vi "Row-Col Average for 2D array.vi"(10 "2D Array":dbl[][](array[numeric])) -> (1 "Column Averages":dbl[](array[numeric]), 2 "Row Averages":dbl[](array[numeric]))   [LabVIEW 2018]
panel:
  out "Total Array Average":dbl
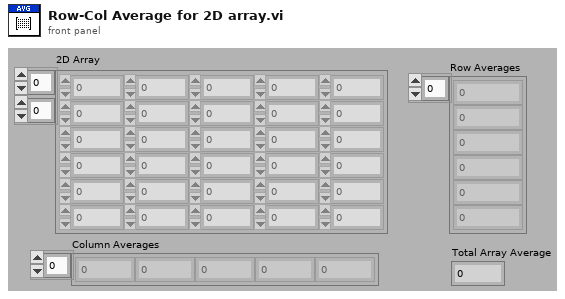
[diagram p1: front panel]
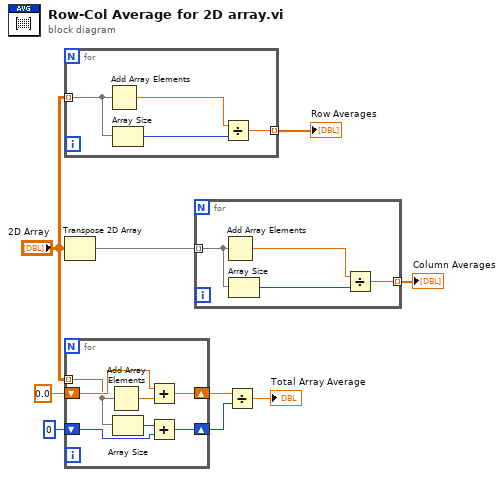
[diagram p0: block diagram]
diagram:
  n1 = for {
    tunnel: "2D Array" -> [w10] mode=indexing
    tunnel: [w12] -> w9 mode=indexing
    n2 = Add Array Elements(numeric array=w10) -> (sum=w13:dbl)
    n3 = Array Size(array=w10) -> (size(s)=w11:i32)
    n4 = Divide(x=w13, y=w11) -> (x/y=w12:dbl)
  }
  "Row Averages" <- w9
  n5 = Transpose 2D Array(2D array="2D Array") -> (transposed array=w8:dbl[][])
  n6 = for {
    tunnel: "2D Array" -> [w17] mode=indexing
    shift-right: [w18] -> w4
    shift-left: 0.0 -> [w20]
    shift-right: [w15] -> w3
    shift-left: 0 -> [w14]
    n7 = Add Array Elements(numeric array=w17) -> (sum=w19:dbl)
    n8 = Array Size(array=w17) -> (size(s)=w16:i32)
    n9 = Add(x=w20, y=w19) -> (x+y=w18:dbl)
    n10 = Add(x=w16, y=w14) -> (x+y=w15:i32)
  }
  n11 = for {
    tunnel: w8 -> [w22] mode=indexing
    tunnel: [w23] -> w7 mode=indexing
    n12 = Add Array Elements(numeric array=w22) -> (sum=w24:dbl)
    n13 = Array Size(array=w22) -> (size(s)=w21:i32)
    n14 = Divide(x=w24, y=w21) -> (x/y=w23:dbl)
  }
  "Column Averages" <- w7
  n15 = Divide(x=w4, y=w3) -> (x/y=→"Total Array Average":dbl)
